vi "_TEST2.vi"() -> ()   [LabVIEW 2019, in "lv-apt-json-file.lvlib"]
uses:
  lv-apt-json-file.lvlib
  Def-AttrMap -- Map.ctl
  612d7cb0-b7e4-4b2c-a714-07072eefdd73.vi
  ef6bff6c-40b4-4ce1-9384-ea178e31dc85.vi
  612d7cb0-b7e4-4b2c-a714-07072eefdd73.vi/8a6843ea-2178-43bd-8e50-deead5b06599.vi
  _Support/AttrMap-SetValue-CORE.vi
  ef6bff6c-40b4-4ce1-9384-ea178e31dc85.vi/7cee1336-6ab3-4b03-8152-783f05cba222.vi
  ef6bff6c-40b4-4ce1-9384-ea178e31dc85.vi/4afbc719-1ad6-49a6-b3e2-32db7922e688.vi
  _Support/AttrMap-SetValue-CORE.vi/6e91e2cf-a420-477d-bf86-627245081caf.vi
  _Support/AttrMap-UnpackMap.vi
  <userlib>/_OpenG.lib/lvdata/lvdata.llb/Get TDEnum from Data__ogtk.vi
panel:
  out "Map":T1
  out "OrgKey String 2":string
  out "found":bool
  out "Value":variant
  out "OrgKey String":string
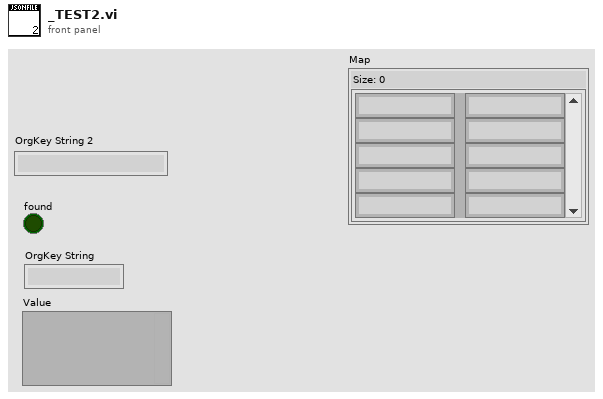
[diagram p1: front panel]
types:
  T1 = typedef "lv-apt-json-file.lvlib/Def-AttrMap -- Map.ctl" = map{string, string}
  T2 = typedef "lv-apt-json-file.lvlib/Def-AttrMap.ctl" = cluster{"Map":variant}
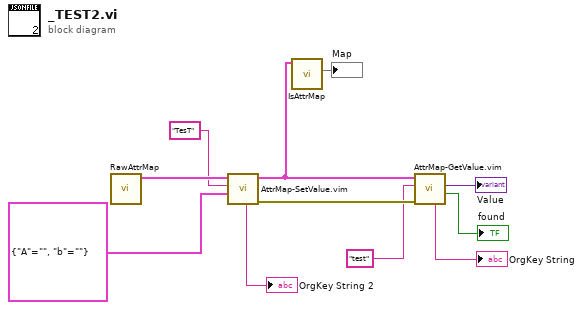
[diagram p0: block diagram]
diagram:
  n1 = call "RawAttrMap.vi"() -> ("AttrMap"=w10:T2)  [unwired: 11 in]
  n2 = call "AttrMap-SetValue.vim"("Value"=cluster{"A":string, "b":string} {"A"="", "b"=""}, "Key(String/Enum)"="TesT", "AttrMap in"=w10) -> ("error out"=w11:errorcluster, "AttrMap out"=w2:T2, "OrgKey String"=→"OrgKey String 2":string)  [unwired: 6 in]
  n3 = call "IsAttrMap.vi"("Variant"=w2) -> ("KeyMap"=→"Map":T1)  [unwired: 8 in, 2 out]
  n4 = call "AttrMap-GetValue.vim"("error in (no error)"=w11, "Key(String/Enum)"="test", "AttrMap in"=w2) -> ("found"=→"found":bool, "Value"=→"Value":variant, "OrgKey String"=→"OrgKey String":string)  [unwired: 4 in, 2 out]
